vi "returns zero connections test.vi"(8 "error in":errorcluster) -> (0 "error out":errorcluster, 2 "result":string, 3 "pass":bool)   [LabVIEW 2020, in "MeasurementServerTests.lvlib"]
uses:
  MeasurementServerTests.lvlib
  Runtime/MeasurementLink Session Management/Session Reservation/Connection.ctl
  Runtime/MeasurementLink Session Management/Session Reservation/Session Reservation.lvclass
  Runtime/MeasurementLink Session Management/Session Reservation/Connection with Session.ctl
  c3cb69a0-23cd-49fc-99d1-8c54773f0200.vi
  Runtime/MeasurementLink Measurement Server/Helpers/Error Strings Global Internal.vi
  Runtime/MeasurementLink niDCPower/Instrument/Instrument.lvclass
  Runtime/MeasurementLink Session Management/Session Reservation/Pin Type.ctl
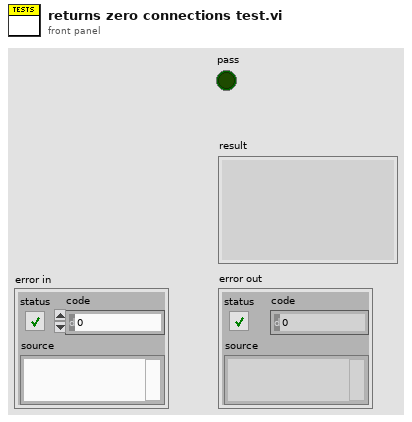
[diagram p1: front panel]
types:
  T1 = typedef "MeasurementLink Session Management.lvlib/Session Reservation.lvclass/Pin Type.ctl" = enum16{"DUT and System Pins", "System Pins"}
  T2 = typedef "MeasurementLink Session Management.lvlib/Session Reservation.lvclass/Connection with Session.ctl" = cluster{"connection":T3, "session":variant}
  T3 = typedef "MeasurementLink Session Management.lvlib/Session Reservation.lvclass/Connection.ctl" = cluster{"pin or relay name":string, "site":i32, "instrument type id":string, "channel":string}
  T4 = typedef "MeasurementLink Session Management.lvlib/Session Reservation.lvclass/Data.ctl" = cluster{"session and driver infos":T5[], "pin or relay names":string[], "connection map":refnum<class "Connection Map.lvclass">, "pin map context":T9, "reservation observer":refnum<class "IReservationObserver.lvclass">, "dvr valid":bool}
  T5 = typedef "MeasurementLink Session Management.lvlib/Session Reservation.lvclass/Session and Driver Info.ctl" = cluster{"session info":T6, "session":variant, "instrument":refnum<class "IInstrument.lvclass">}
  T6 = typedef "MeasurementLink Session Management Client.lvlib/ni_measurementlink_sessionmanagement_v1_SessionInformation.ctl" = cluster{"session":T7, "resource_name":string, "channel_list":string, "instrument_type_id":string, "session_exists":bool, "channel_mappings":T8[]}
  T7 = typedef "MeasurementLink Session Management Client.lvlib/nidevice_grpc_Session.ctl" = cluster{"name":string}
  T8 = typedef "MeasurementLink Session Management Client.lvlib/ni_measurementlink_sessionmanagement_v1_ChannelMapping.ctl" = cluster{"pin_or_relay_name":string, "site":i32, "channel":string}
  T9 = typedef "MeasurementLink Session Management Client.lvlib/ni_measurementlink_PinMapContext.ctl" = cluster{"pin_map_id":string, "sites":i32[]}
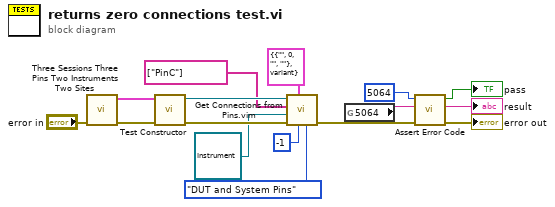
[diagram p0: block diagram]
diagram:
  n1 = call "Three Sessions Three Pins Two Instruments Two Sites.vi"("error in"="error in") -> ("error out"=w11:errorcluster, "data out"=w10:T4)  [unwired: 9 in]
  n2 = call "Test Constructor.vi"("error in"=w11, "data"=w10) -> ("error out"=w15:errorcluster, "Session Reservation out"=w14:refnum<class "Session Reservation.lvclass">)  [unwired: 8 in]
  n3 = call "Get Connections from Pins.vim"("pin type"=Pin_Type."DUT and System Pins", "site"=-1, "connection type"=T2 {"connection"={"pin or relay name"="", "site"=0, "instrument type id"="", "channel"=""}, "session"=variant} ("connection"), "error in"=w15, "instrument"=refnum<class "Instrument.lvclass"> refnum ("MeasurementLink niDCPower.lvlib:Instrument.lvclass"), "pin or relay names"=string[] ["PinC"], "session reservation in"=w14) -> ("error out"=w6:errorcluster)  [unwired: 2 in, 2 out]
  n4 = global read "Error Strings Global Internal.vi" "5064"() -> (w7:string)
  n5 = call "Assert Error Code.vi"("error in"=w6, "expected error description"=w7, "expected error code"=5064) -> ("error out"=→"error out":errorcluster, "details"=→"result":string, "error code match?"=→"pass":bool)  [unwired: 6 in]
